vi "Hysteresis_min.vi"(0 "input":dbl, 5 "Min":dbl=26.0 format="%#_13g", 7 "H":dbl=22.0 format="%#_13g", 11 "error in":errorcluster) -> (8 "Deviation":bool, 15 "error out":errorcluster)   [LabVIEW 2022 SP3]
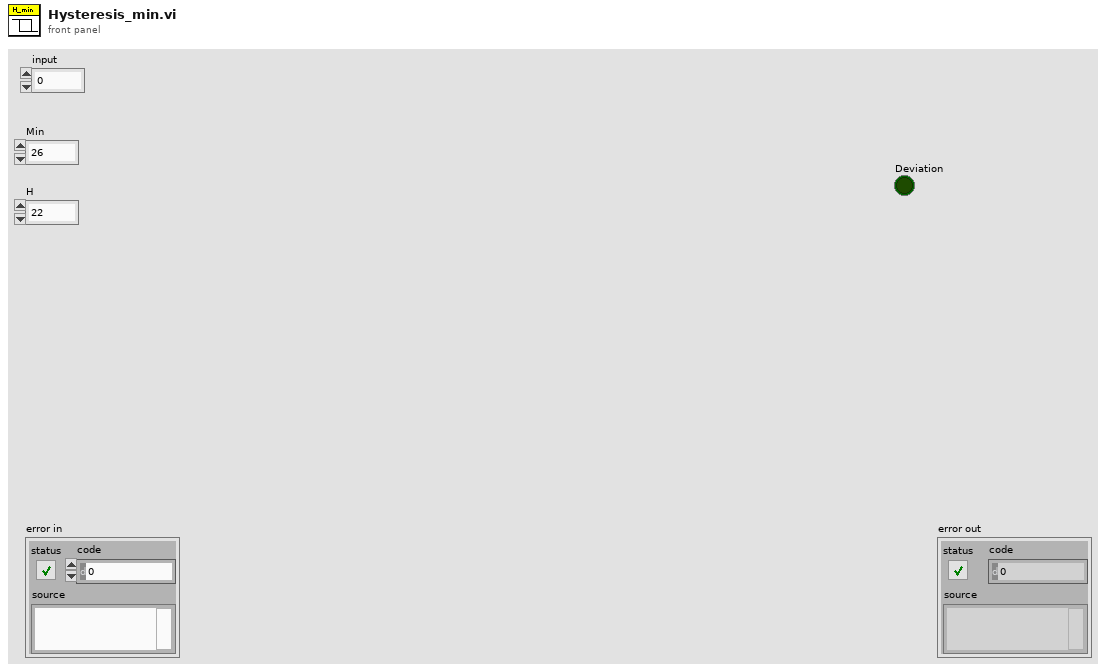
[diagram p1: front panel]
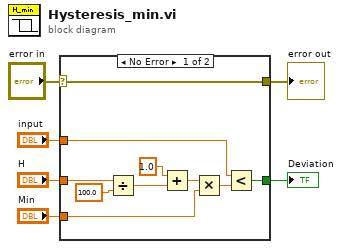
[diagram p0: block diagram]
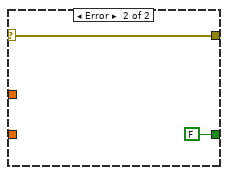
[diagram p2: hidden frame]
diagram:
  n1 = case shown="No Error" "error in" {
    selector: "error in" -> [w9 w18]
    tunnel: "H" -> [w12 _]
    tunnel: "input" -> [w11 _]
    tunnel: "Min" -> [w10 _]
    tunnel: [w9 w18] -> w2
    tunnel: [w8 FALSE] -> w1
    frame No Error {
      n2 = Divide(x=w12, y=100.0) -> (x/y=w16:dbl)
      n3 = Add(x=1.0 ("y"), y=w16) -> (x+y=w13:dbl)
      n4 = Multiply(x=w13, y=w10) -> (x*y=w7:dbl)
      n5 = Less?(x=w11, y=w7) -> (x < y?=w8:bool)
    }
    frame Error {
    }
  }
  "error out" <- w2
  "Deviation" <- w1
